vi "CVT String Write.vi"(3 "error in (no error)":errorcluster, 4 "Value":string, 5 "Tag Name":string) -> (0 "error out":errorcluster)   [LabVIEW 2010]
uses:
  _SubVIs/TypeDefs/cvt_MemBlock Methods.ctl
  _SubVIs/TypeDefs/cvt_TagList Methods.ctl
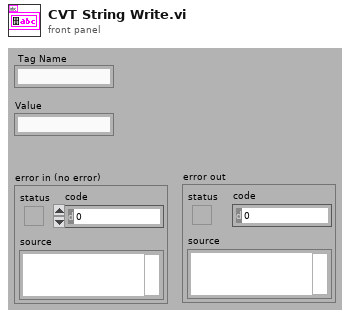
[diagram p1: front panel]
types:
  T1 = typedef "cvt_MemBlock Methods.ctl" = enum16{"init", "read", "readall", "write"}
  T2 = typedef "cvt_TagList Methods.ctl" = enum16{"init", "getindex", "getdesc", "getlist"}
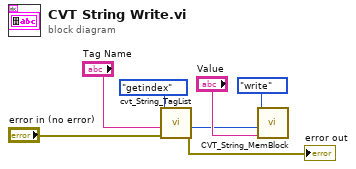
[diagram p0: block diagram]
diagram:
  n1 = call "cvt_String_TagList.vi"("error in (no error)"="error in (no error)", "Tag Name"="Tag Name", "Method"=cvt_TagList_Methods."getindex") -> ("error out"=→"error out":errorcluster, "Index"=w5:i32)  [unwired: 1 in, 6 out]
  n2 = call "CVT_String_MemBlock.vi"("Value"="Value", "Index"=w5, "Method"=cvt_MemBlock_Methods."write") -> ()  [unwired: 1 in, 8 out]
